vi "createPubDataEvents.vi"(8 "error in (no error)":errorcluster, 11 "UserEvents in":refnum<class "UserEvents.lvclass">) -> (0 "error out":errorcluster, 3 "UserEvents out":refnum<class "UserEvents.lvclass">)   [LabVIEW 2013, in "UserEvents.lvclass"]
uses:
  UserEvents.lvclass
  Typedefs/StateSelector.ctl
  Typedefs/InputData.ctl
  <userlib>/Common/ILC/Typedefs/LimitSwitches.ctl
  Typedefs/ForceDemand.ctl
  <userlib>/Common/Devices/DistanceGauge/Typedefs/Distance Data.ctl
  Typedefs/ThermocoupleData.ctl
  Typedefs/OutputData.ctl
  Typedefs/ControllerData.ctl
  Typedefs/TestStatus.ctl
  Typedefs/StiffnessData.ctl
  UserEvents.lvclass/UserEvents.ctl
  Typedefs/M2AADTTypedefs.lvlib
  <userlib>/Common/ILC/Typedefs/ILCTypedefs.lvlib
  <userlib>/Common/Devices/DistanceGauge/DistanceGauge.lvlib
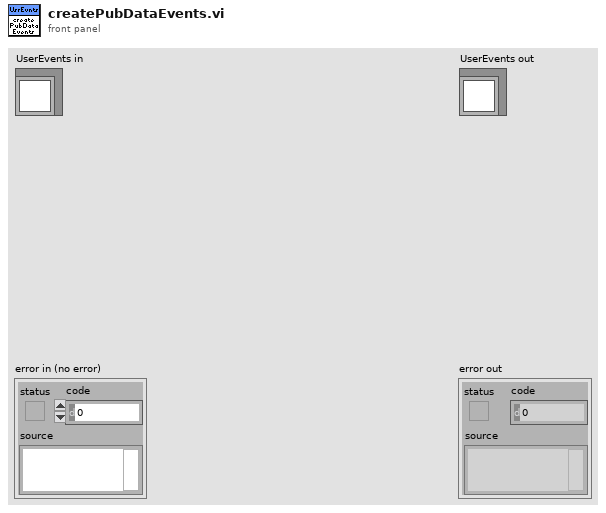
[diagram p1: front panel]
types:
  T1 = typedef "M2AADTTypedefs.lvlib/StiffnessData.ctl" = cluster{"Constrained Displacement":dbl[unit], "Stiffness":dbl[unit]}
  T2 = typedef "M2AADTTypedefs.lvlib/TestStatus.ctl" = cluster{"activeCycle":u32, "activeProfileStep":u32, "demandedCycles":u32, "demandedProfileSteps":u32}
  T3 = typedef "M2AADTTypedefs.lvlib/ControllerData.ctl" = cluster{"Force Demand":T4, "Force Error":T4}
  T4 = typedef "M2AADTTypedefs.lvlib/ForceDemand.ctl" = dbl[unit]
  T5 = typedef "M2AADTTypedefs.lvlib/OutputData.ctl" = cluster{"Step & Direction":i16}
  T6 = typedef "M2AADTTypedefs.lvlib/InputData.ctl" = cluster{"Limit Switches":T7, "SSI Encoder":i32, "Force Measured":T4, "Distance Data":T8, "Thermocouple Data":T9}
  T7 = typedef "ILCCommon.lvlib/ILCTypedefs.lvlib/LimitSwitches.ctl" = cluster{"1":bool, "2":bool}
  T8 = typedef "DistanceGauge.lvlib/Distance Data.ctl" = cluster{"Distance Measured 1":dbl[unit], "Distance Measured 2":dbl[unit]}
  T9 = typedef "M2AADTTypedefs.lvlib/ThermocoupleData.ctl" = cluster{"Motor Temperature":dbl[unit]}
  T10 = typedef "M2AADTTypedefs.lvlib/StateSelector.ctl" = enum16{"EndingCycleState", "FaultState", "InteractiveMotionState", "MovingToNewForceState", "OffState", "PausingState", "StandbyState", "StoppedState"}
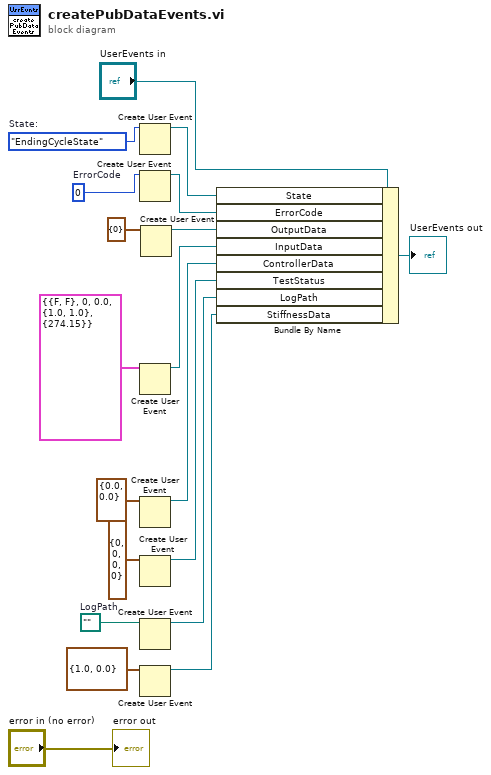
[diagram p0: block diagram]
diagram:
  w4 = path ""  # LogPath
  w15 = 0  # ErrorCode
  w16 = StateSelector."EndingCycleState"  # State:
  n1 = Create User Event(user event datatype=w16) -> (user event=w14:refnum<user-event>)  [unwired: 1 in, 1 out]
  n2 = Create User Event(user event datatype=w15) -> (user event=w13:refnum<user-event>)  [unwired: 1 in, 1 out]
  n3 = Create User Event(user event datatype=T6 {"Limit Switches"={"1"=FALSE, "2"=FALSE}, "SSI Encoder"=0, "Force Measured"=0.0, "Distance Data"={"Distance Measured 1"=1.0, "Distance Measured 2"=1.0}, "Thermocouple Data"={"Motor Temperature"=274.15}} ("Input Data")) -> (user event=w11:refnum<user-event>)  [unwired: 1 in, 1 out]
  n4 = Create User Event(user event datatype=T3 {"Force Demand"=0.0, "Force Error"=0.0} ("Controller Data")) -> (user event=w7:refnum<user-event>)  [unwired: 1 in, 1 out]
  n5 = Create User Event(user event datatype=T2 {"activeCycle"=0, "activeProfileStep"=0, "demandedCycles"=0, "demandedProfileSteps"=0} ("TestStatus")) -> (user event=w5:refnum<user-event>)  [unwired: 1 in, 1 out]
  n6 = Create User Event(user event datatype=w4) -> (user event=w3:refnum<user-event>)  [unwired: 1 in, 1 out]
  n7 = Create User Event(user event datatype=T1 {"Constrained Displacement"=1.0, "Stiffness"=0.0} ("output cluster")) -> (user event=w1:refnum<user-event>)  [unwired: 1 in, 1 out]
  n8 = Create User Event(user event datatype=T5 {"Step & Direction"=0} ("Output Data")) -> (user event=w9:refnum<user-event>)  [unwired: 1 in, 1 out]
  n9 = Bundle By Name(cluster="UserEvents in", "State"=w14, "ErrorCode"=w13, "OutputData"=w9, "InputData"=w11, "ControllerData"=w7, "TestStatus"=w5, "LogPath"=w3, "StiffnessData"=w1) -> (→"UserEvents out":refnum<class "UserEvents.lvclass">)
  "error out" <- "error in (no error)"
